vi "Rotate_DBL.vi"(7 "Direction of Rotation":T1, 8 "error in (no error)":errorcluster, 10 "Angle (degrees)":dbl, 11 "CartesianVector in":refnum<class "CartesianVector.lvclass">) -> (0 "error out":errorcluster, 3 "CartesianVector out":refnum<class "CartesianVector.lvclass">)   [LabVIEW 2011, in "CartesianVector.lvclass"]
uses:
  CartesianVector.lvclass
  TypeDefs/DirectionOfRotation.ctl
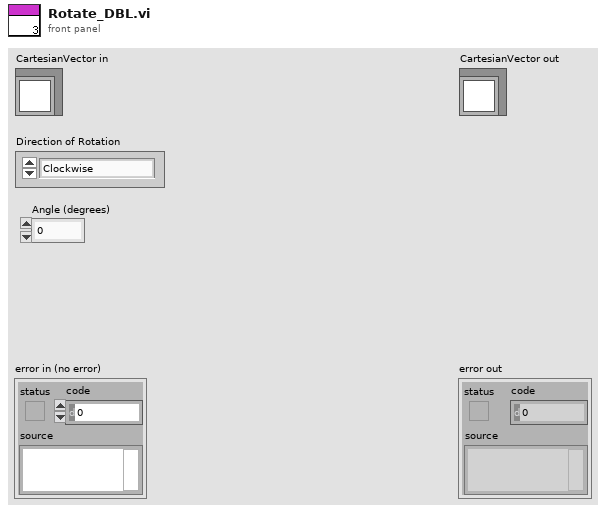
[diagram p1: front panel]
types:
  T1 = typedef "DirectionOfRotation.ctl" = enum16{"Clockwise", "Counter-Clockwise"}
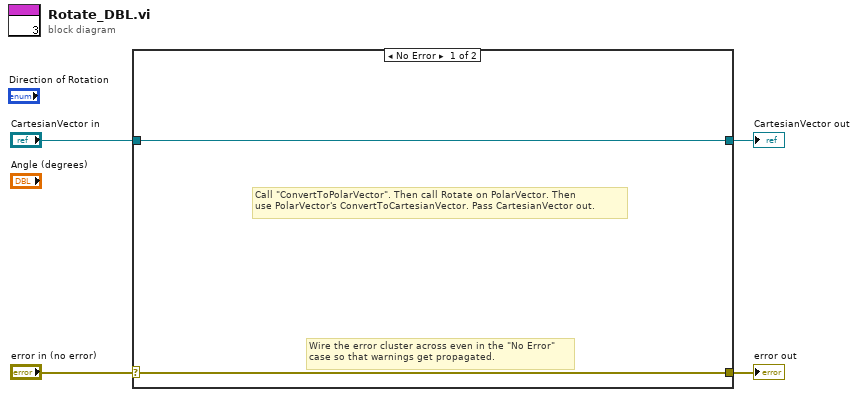
[diagram p0: block diagram]
diagram:
  n1 = case shown="No Error" "error in (no error)" {
    selector: "error in (no error)" -> [w5 w8]
    tunnel: [w5 w8] -> w3
    tunnel: [w6 w7] -> w1
    tunnel: "CartesianVector in" -> [w6 w7]
    frame No Error {
      # "Call \"ConvertToPolarVector\". Then call Rotate on PolarVector. Then\nuse PolarVector's ConvertToCartesianVector. Pass CartesianVector out."
      # "Wire the error cluster across even in the \"No Error\"\ncase so that warnings get propagated."
    }
    frame Error {
    }
  }
  "error out" <- w3
  "CartesianVector out" <- w1
